vi "Move Tool Diagnostics Section.vi"(8 "error in (no error)":errorcluster, 11 "Device Item Ref in":T1 format="%.0x") -> (0 "error out":errorcluster, 3 "Device Item Ref Out":T1=18446744073709551615 format="%.0x")   [LabVIEW 2023, in "J1939 Addon System Explorer.lvlib"]
uses:
  J1939 Addon System Explorer.lvlib
  <vilib>/NI VeriStand/Custom Device API/Custom Device Item Ref.ctl
  <vilib>/NI VeriStand/Custom Device API/Custom Device Channel.ctl
  <vilib>/NI VeriStand/Custom Device API/Custom Device Channel Type.ctl
  Addon Shared/SubVIs/Constants.vi
  <vilib>/NI VeriStand/Custom Device API/Custom Device API.lvlib
  Addon Shared/J1939 Addon Shared.lvlib
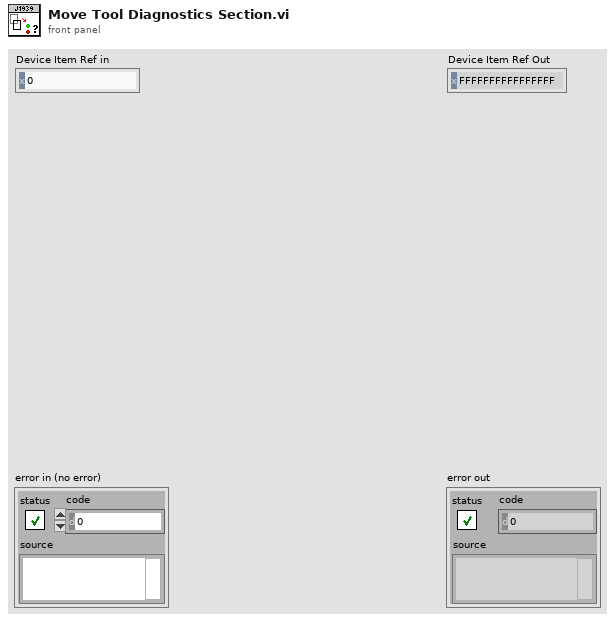
[diagram p1: front panel]
types:
  T1 = typedef "Custom Device API.lvlib/Custom Device Item Ref.ctl" = u64
  T2 = typedef "Custom Device API.lvlib/Custom Device Channel.ctl" = cluster{"Type":T3, "Units":string, "Default Value":dbl, "Faultable":bool, "Scalable":bool}
  T3 = typedef "Custom Device API.lvlib/Custom Device Channel Type.ctl" = enum16{"Input", "Output"}
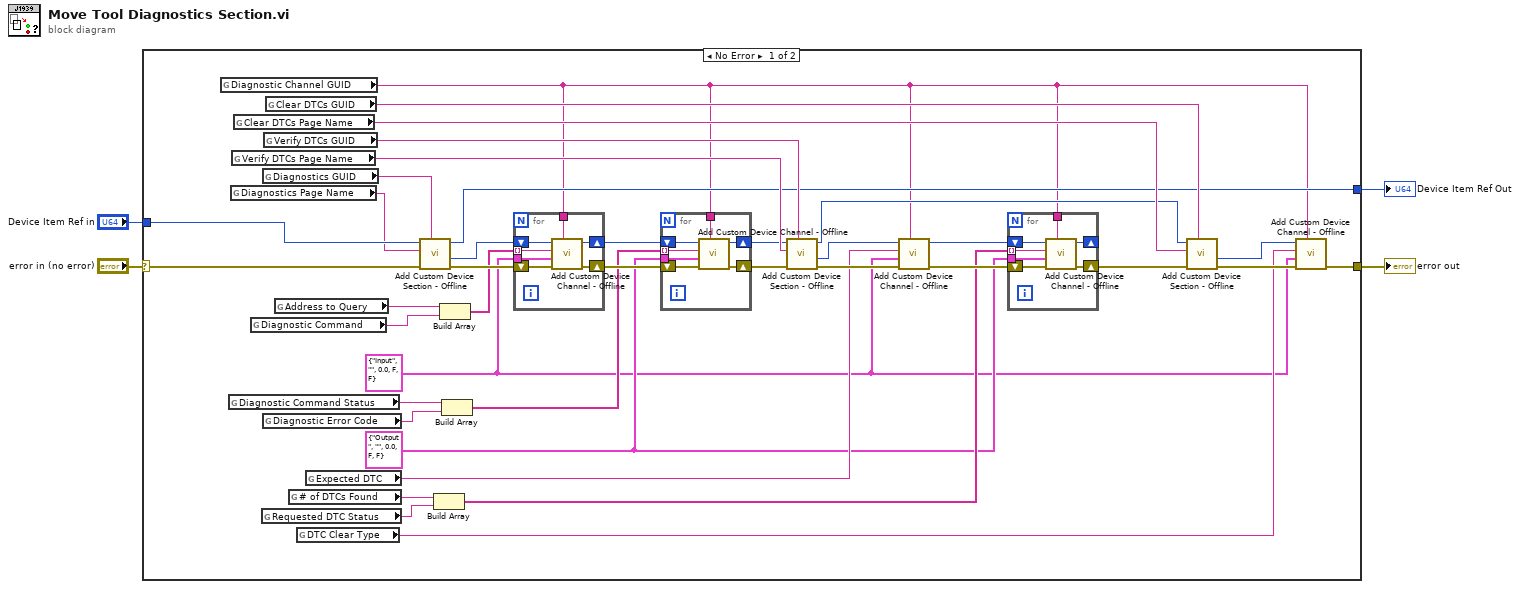
[diagram p0: block diagram]
diagram:
  n1 = case shown="No Error" "error in (no error)" {
    selector: "error in (no error)" -> [w41 w65]
    tunnel: [w12 w65] -> w3
    tunnel: "Device Item Ref in" -> [w42 w64]
    tunnel: [w8 w64] -> w1
    frame No Error {
      w7 = T2 {"Type"=enum."Output", "Units"="", "Default Value"=0.0, "Faultable"=FALSE, "Scalable"=FALSE} ("Channel")
      w6 = T2 {"Type"=enum."Input", "Units"="", "Default Value"=0.0, "Faultable"=FALSE, "Scalable"=FALSE} ("Channel")
      n2 = global read "Constants.vi" "Diagnostic Channel GUID"() -> (w5:string)
      n3 = global read "Constants.vi" "Diagnostic Command Status"() -> (w27:string)
      n4 = global read "Constants.vi" "Diagnostics Page Name"() -> (w39:string)
      n5 = global read "Constants.vi" "Verify DTCs Page Name"() -> (w37:string)
      n6 = global read "Constants.vi" "Clear DTCs Page Name"() -> (w15:string)
      n7 = global read "Constants.vi" "Diagnostic Command"() -> (w33:string)
      n8 = global read "Constants.vi" "Requested DTC Status"() -> (w18:string)
      n9 = global read "Constants.vi" "Diagnostics GUID"() -> (w40:string)
      n10 = global read "Constants.vi" "Diagnostic Error Code"() -> (w26:string)
      n11 = global read "Constants.vi" "Verify DTCs GUID"() -> (w38:string)
      n12 = global read "Constants.vi" "Clear DTCs GUID"() -> (w14:string)
      n13 = global read "Constants.vi" "Address to Query"() -> (w34:string)
      n14 = global read "Constants.vi" "# of DTCs Found"() -> (w19:string)
      n15 = global read "Constants.vi" "DTC Clear Type"() -> (w10:string)
      n16 = global read "Constants.vi" "Expected DTC"() -> (w20:string)
      n17 = call "Add Custom Device Section - Offline.vi"("GUID (Default Section)"=w40, "error in (no error)"=w41, "Section Name"=w39, "Parent Ref in"=w42) -> ("error out"=w36:errorcluster, "Section Ptr"=w35:T1, "Parent Ref out"=w8:T1)  [unwired: 4 in, 1 out]
      n18 = Build Array(w19, w18) -> (w17:string[])
      n19 = Build Array(w34, w33) -> (w32:string[])
      n20 = Build Array(w27, w26) -> (w25:string[])
      n21 = for {
        tunnel: w32 -> [w59] mode=indexing
        shift-right: [w60] -> w30
        shift-left: w35 -> [w61]
        shift-right: [w62] -> w31
        shift-left: w36 -> [w63]
        tunnel: w6 -> [w58]
        tunnel: w5 -> [w57]
        n22 = call "Add Custom Device Channel - Offline.vi"("GUID (Default Channel)"=w57, "error in (no error)"=w63, "Channel"=w58, "Channel Name"=w59, "Parent Ref in"=w61) -> ("error out"=w62:errorcluster, "Parent Ref out"=w60:T1)  [unwired: 3 in, 2 out]
      }
      n23 = for {
        tunnel: w25 -> [w52] mode=indexing
        shift-right: [w53] -> w28
        shift-left: w30 -> [w54]
        shift-right: [w55] -> w29
        shift-left: w31 -> [w56]
        tunnel: w7 -> [w51]
        tunnel: w5 -> [w50]
        n24 = call "Add Custom Device Channel - Offline.vi"("GUID (Default Channel)"=w50, "error in (no error)"=w56, "Channel"=w51, "Channel Name"=w52, "Parent Ref in"=w54) -> ("error out"=w55:errorcluster, "Parent Ref out"=w53:T1)  [unwired: 3 in, 2 out]
      }
      n25 = call "Add Custom Device Section - Offline.vi"("GUID (Default Section)"=w38, "error in (no error)"=w29, "Section Name"=w37, "Parent Ref in"=w28) -> ("error out"=w22:errorcluster, "Section Ptr"=w24:T1, "Parent Ref out"=w9:T1)  [unwired: 4 in, 1 out]
      n26 = call "Add Custom Device Channel - Offline.vi"("GUID (Default Channel)"=w5, "error in (no error)"=w22, "Channel"=w6, "Channel Name"=w20, "Parent Ref in"=w24) -> ("error out"=w23:errorcluster, "Parent Ref out"=w21:T1)  [unwired: 3 in, 2 out]
      n27 = for {
        tunnel: w17 -> [w45] mode=indexing
        shift-right: [w46] -> _
        shift-left: w21 -> [w47]
        shift-right: [w48] -> w16
        shift-left: w23 -> [w49]
        tunnel: w7 -> [w44]
        tunnel: w5 -> [w43]
        n28 = call "Add Custom Device Channel - Offline.vi"("GUID (Default Channel)"=w43, "error in (no error)"=w49, "Channel"=w44, "Channel Name"=w45, "Parent Ref in"=w47) -> ("error out"=w48:errorcluster, "Parent Ref out"=w46:T1)  [unwired: 3 in, 2 out]
      }
      n29 = call "Add Custom Device Section - Offline.vi"("GUID (Default Section)"=w14, "error in (no error)"=w16, "Section Name"=w15, "Parent Ref in"=w9) -> ("error out"=w13:errorcluster, "Section Ptr"=w11:T1)  [unwired: 4 in, 2 out]
      n30 = call "Add Custom Device Channel - Offline.vi"("GUID (Default Channel)"=w5, "error in (no error)"=w13, "Channel"=w6, "Channel Name"=w10, "Parent Ref in"=w11) -> ("error out"=w12:errorcluster)  [unwired: 3 in, 3 out]
    }
    frame Error {
    }
  }
  "error out" <- w3
  "Device Item Ref Out" <- w1
